vi "Send Message.vi"(8 "error in (no error)":errorcluster, 10 "Messaje":string, 11 "Message Actor in":refnum<class "Message Actor.lvclass">) -> (0 "error out":errorcluster, 3 "Message Actor out":refnum<class "Message Actor.lvclass">)   [LabVIEW 2020, in "Message Actor.lvlib" / "Message Actor.lvclass"]
uses:
  Message Actor.lvclass
  Message Actor.lvclass/Message Actor.ctl
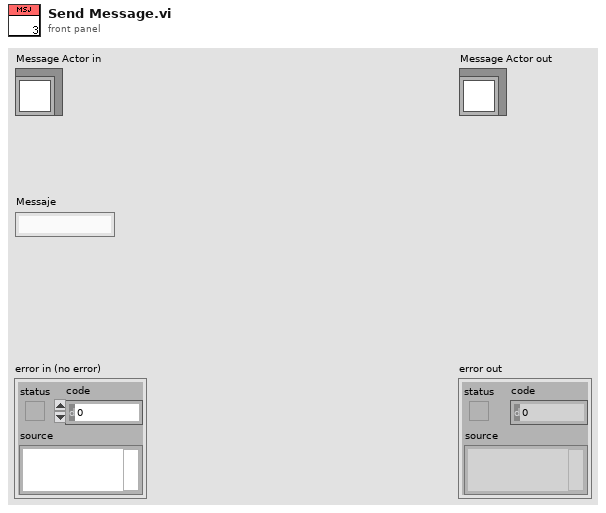
[diagram p1: front panel]
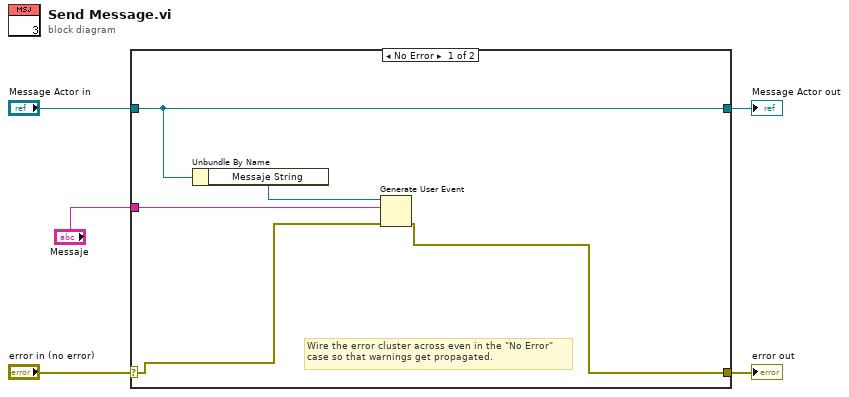
[diagram p0: block diagram]
diagram:
  n1 = case shown="No Error" "error in (no error)" {
    selector: "error in (no error)" -> [w6 w12]
    tunnel: [w7 w12] -> w4
    tunnel: [w10 w11] -> w2
    tunnel: "Message Actor in" -> [w10 w11]
    tunnel: "Messaje" -> [w8 _]
    frame No Error {
      # "Wire the error cluster across even in the \"No Error\"\ncase so that warnings get propagated."
      n2 = Unbundle By Name(w10) -> ("Messaje String"=w9:refnum<user-event>)
      n3 = Generate User Event(user event=w9, event data cluster=w8, error in=w6) -> (error out=w7:errorcluster)  [unwired: 1 in, 1 out]
    }
    frame Error {
    }
  }
  "error out" <- w4
  "Message Actor out" <- w2
